vi "FileList.vi"(8 "error in (no error)":errorcluster, 11 "controller in":refnum<k24>) -> (0 "error out":errorcluster, 1 "Number of Files":i32, 2 "File List":T1(array[cluster]), 3 "controller out":refnum<k24>)   [LabVIEW 2010]
uses:
  c:/aerotech/controller/5.xx.xxx/ensemble/pc/labview/2010/bin/Aerotech.Ensemble.dll
  bin/Aerotech.Ensemble.dll
  c:/aerotech/controller/5.xx.xxx/ensemble/pc/labview/2010/bin/Aerotech.Ensemble.LabVIEW.dll
  bin/Aerotech.Ensemble.LabVIEW.dll
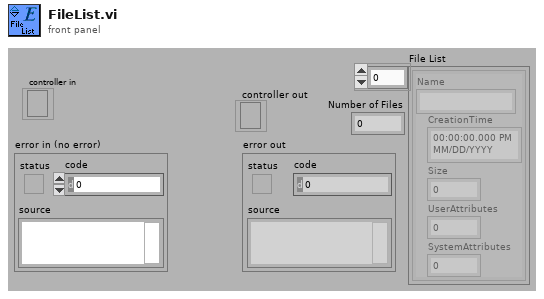
[diagram p1: front panel]
types:
  T1 = cluster{"Name":string, "CreationTime":timestamp, "Size":i32, "UserAttributes":i32, "SystemAttributes":i32}[]
  T2 = cluster{"Name":string, "CreationTime":timestamp, "Size":i32, "UserAttributes":i32, "SystemAttributes":i32}
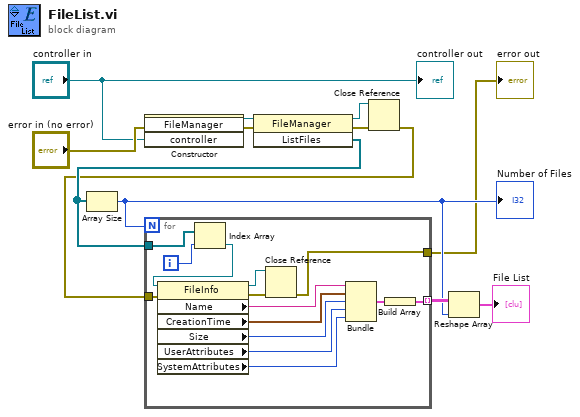
[diagram p0: block diagram]
diagram:
  n1 = constructor class="FileManager"(error in="error in (no error)", "controller"="controller in") -> (reference out=w7:refnum<k24>, error out=w9:errorcluster)  [unwired: 2 in, 2 out]
  n2 = invoke class="FileManager" method="ListFiles"(reference=w7, error in=w9) -> (reference out=w11:refnum<k24>, error out=w12:errorcluster, "ListFiles"=w6:refnum<k24>[])  [unwired: 1 in]
  n3 = Array Size(array=w6) -> (size(s)=w3:i32)
  "Number of Files" <- w3
  n4 = Close Reference(reference=w11, error in (no error)=w12) -> (error out=w2:errorcluster)
  n5 = for {
    N: w3 -> [_]
    tunnel: w6 -> [w20]
    tunnel: [w19] -> w5 mode=indexing
    tunnel: w2 -> [w16]
    tunnel: [w13] -> w1
    i -> [w21]
    n6 = Index Array(array=w20, index=w21) -> (element=w17:refnum<k24>)
    n7 = property class="FileInfo"(reference=w17, error in=w16) -> (reference out=w14:refnum<k24>, error out=w15:errorcluster, "Name"=w26:string, "CreationTime"=w25:timestamp, "Size"=w24:i32, "UserAttributes"=w23:i32, "SystemAttributes"=w22:i32)
    n8 = Close Reference(reference=w14, error in (no error)=w15) -> (error out=w13:errorcluster)
    n9 = Bundle("Name"=w26, "CreationTime"=w25, "Size"=w24, "UserAttributes"=w23, "SystemAttributes"=w22) -> (w18:T2)  [unwired: 1 in]
    n10 = Build Array(w18) -> (w19:T1)
  }
  "error out" <- w1
  n11 = Reshape Array(w5, w3) -> (→"File List":T1)
  "controller out" <- "controller in"
